vi "GetLayerQTY.vi"(8 "error in (no error)":errorcluster, 11 "FAMM in":refnum<class "FAMM.lvclass">) -> (0 "error out":errorcluster, 1 "FAMM_PAQ_resolution":dbl format="%.3f", 2 "FAMM_PAQ_Layers":i32, 3 "FAMM out":refnum<class "FAMM.lvclass">)   [LabVIEW 2020, in "FAMM.lvclass"]
doc: "Retrieve Layer quantity (6...9) and PAQ acquisition resolution"
uses:
  FAMM.lvclass
  FAMM.lvclass/FAMM.ctl
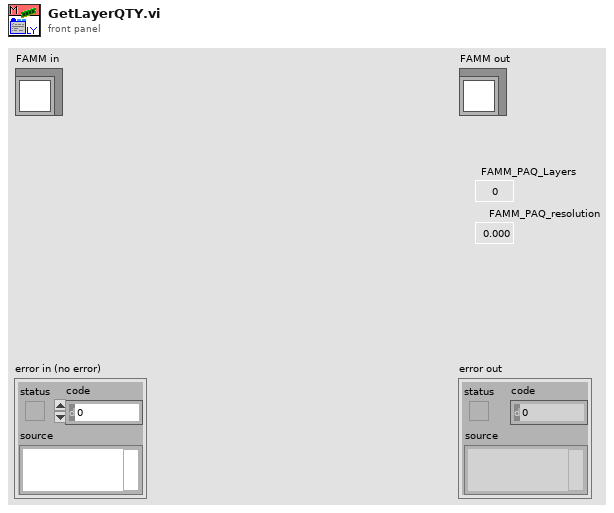
[diagram p1: front panel]
types:
  T1 = typedef "FAMM.lvclass/FAMM-attributes.ctl" = cluster{"FAMM_PAQ_Layers":i32, "FAMM_PAQ_resolution":dbl, "PAQ_TAGs":string[], "WAQ_TAGs":string[], "EAQ_TAGs":string[], "All_TAGs":string[], "PAQtagProps":T2[], "WAQtagProps":T2[], "EAQtagProps":T2[], "DBAL_class":refnum<data-value>, "PAQ_memory":refnum<data-value>[], "PAQupdates":timestamp[], "FAMM_Size":cluster{"other":i32, "1day":i32, "1week":i32}, "DatabaseFileExtention":string, "DatabaseSaveRate":dbl, "Database_path":path}
  T2 = typedef "typedef_com_TagProp.ctl" = cluster{"Description":string, "EngUnits":string, "RangeH":dbl, "RangeL":dbl, "Resolution":i32, "Obsolete":bool, "ChangeDate":timestamp, "ChangeSource":string, "ChangeReason":string, "TagFunc":u32}
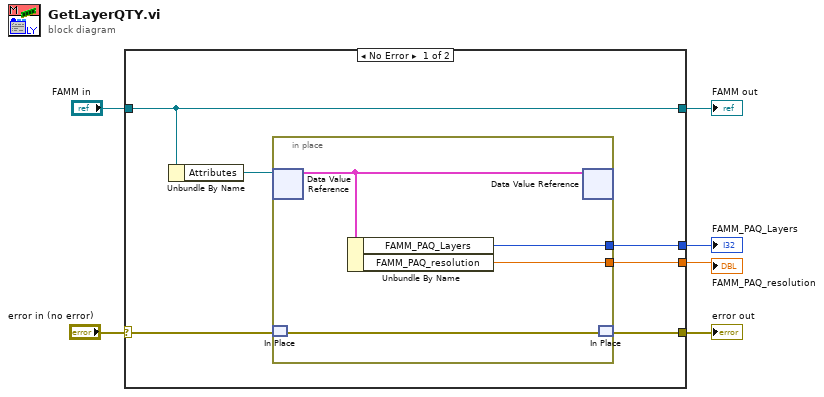
[diagram p0: block diagram]
diagram:
  n1 = case shown="No Error" "error in (no error)" {
    selector: "error in (no error)" -> [w12 w18]
    tunnel: [w11 w18] -> w5
    tunnel: [w8 w17] -> w4
    tunnel: "FAMM in" -> [w8 w17]
    tunnel: [w10 _] -> w3
    tunnel: [w9 _] -> w2
    frame No Error {
      n2 = Unbundle By Name(w8) -> ("Attributes"=w7:refnum<data-value>)
      n3 = in-place {
        in-place-border: [w14] -> w10
        in-place-border: [w13] -> w9
        n4 = in-place-dvr #1(w7) -> (w15:T1)  [unwired: 1 out]
        n5 = in-place-match #2(w12) -> (w16:errorcluster)
        n6 = Unbundle By Name(w15) -> ("FAMM_PAQ_Layers"=w13:i32, "FAMM_PAQ_resolution"=w14:dbl)
        n7 = in-place-dvr #1(w15) -> ()  [unwired: 2 out]
        n8 = in-place-match #2(w16) -> (w11:errorcluster)
      }
    }
    frame Error {
    }
  }
  "error out" <- w5
  "FAMM out" <- w4
  "FAMM_PAQ_Layers" <- w2
  "FAMM_PAQ_resolution" <- w3
